vi "Core Action.vi"(8 "error in (no error)":errorcluster, 10 "SECS-II Class In":refnum<class "SECS-II Class.lvclass">, 11 "33-Update Trace Data in":refnum<class "33-Update Trace Data.lvclass">) -> (0 "error out":errorcluster, 2 "SECS-II Class Out":refnum<class "SECS-II Class.lvclass">, 3 "33-Update Trace Data out":refnum<class "33-Update Trace Data.lvclass">)   [LabVIEW 2020, in "SECS Scenarios.lvlib" / "33-Update Trace Data.lvclass"]
uses:
  33-Update Trace Data.lvclass
  D:/Dropbox/SECS/SECS_GEM v1.1.0/Com/SECS Scenarios/Scenarios Class/Scenarios Class.lvclass
  SECS Communication/SECS-II Class/SECS-II Class.lvclass
  SECS Communication/S6 Message Class/S6 Message Class.lvclass
  D:/Dropbox/SECS/SECS_GEM v1.1.0/Com/SECS Communication/SECS-II Class/SECS-II Class.lvclass
  33-Update Trace Data.lvclass/33-Update Trace Data.ctl
  Scenarios Class/Scenarios Class.lvclass/Scenarios Class.ctl
  Scenarios Class/Reply State.ctl
  Scenarios Class/Write Reply State.vi
  Scenarios Class/Read HSMS Class.vi
  SECS Communication/HSMS Class/HSMS Class.lvclass
  Scenarios Class/Scenarios Class.lvclass
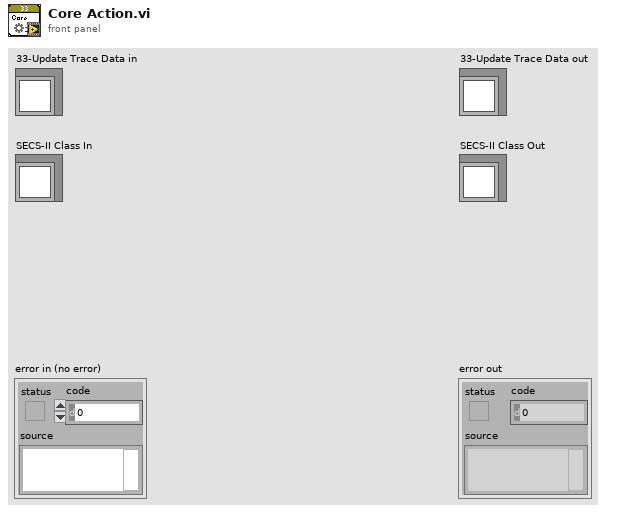
[diagram p1: front panel]
types:
  T1 = typedef "SECS Communication.lvlib/S6 Message Class.lvclass/S6F1.ctl" = cluster{"TRID":u32, "SMPLN":u32, "STIME":string, "SV":cluster{"Format Code":T2, "Value":variant}[]}
  T2 = typedef "SECS Communication.lvlib/SECS-II Class.lvclass/Format Code.ctl" = enum16{"L", "A", "B", "Boolean", "J", "I1", "I2", "I4", "I8", "U1", "U2", "U4", "U8", "F4", "F8", "Char"}
  T3 = typedef "SECS Scenarios.lvlib/Scenarios Class.lvclass/Reply State.ctl" = enum16{"OK", "Illegal Data", "Unknown Stream", "Unknown Function", "Off-Line", "T3 Timeout", "Inner-Timeout"}
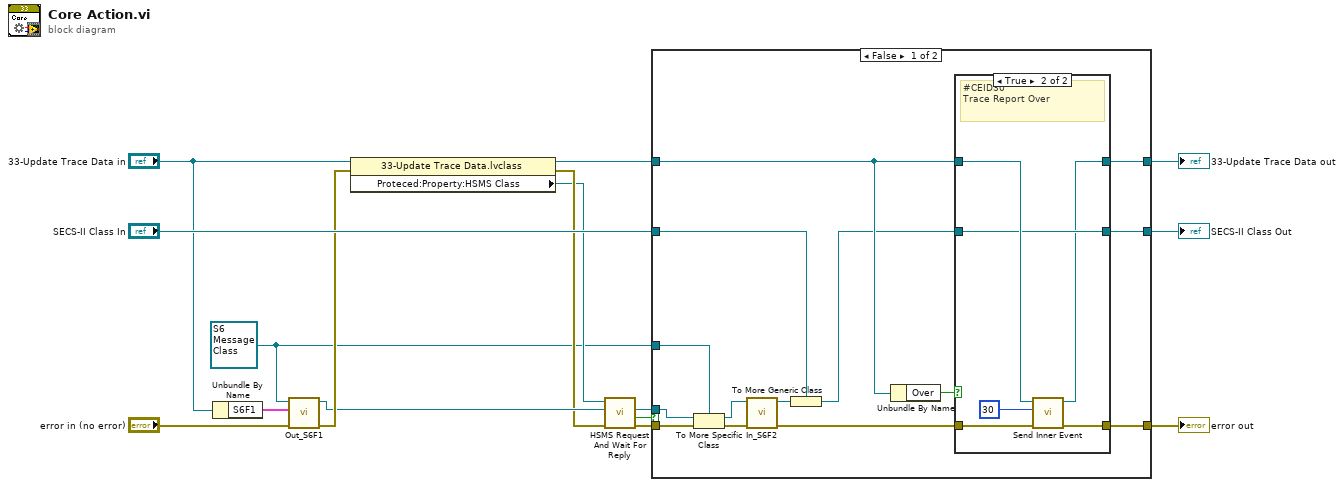
[diagram p0: block diagram]
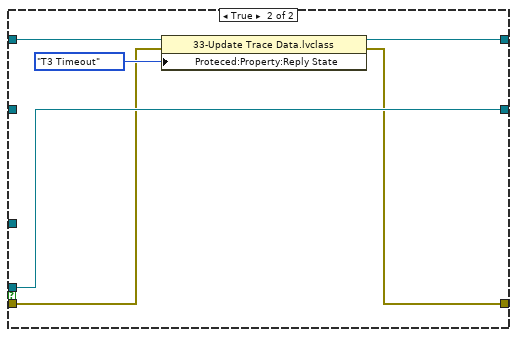
[diagram p3: hidden frame]
diagram:
  w5 = refnum<class "S6 Message Class.lvclass"> refnum ("SECS Communication.lvlib:S6 Message Class.lvclass")
  n1 = Unbundle By Name("33-Update Trace Data in") -> ("S6F1"=w4:T1)
  n2 = call "Out_S6F1.vi"("error in (no error)"="error in (no error)", "S6F1"=w4, "S6 Message Class in"=w5) -> ("error out"=w13:errorcluster, "S6 Message Class out"=w12:refnum<class "S6 Message Class.lvclass">)  [unwired: 7 in]
  n3 = property class="33-Update Trace Data.lvclass"(reference="33-Update Trace Data in", error in=w13) -> (reference out=w6:refnum<class "33-Update Trace Data.lvclass">, error out=w11:errorcluster, "Proteced:Property:HSMS Class"=w10:refnum<class "HSMS Class.lvclass">)
  n4 = call "HSMS Request And Wait For Reply.vi"("error in (no error)"=w11, "SECS-II Class In"=w12, "HSMS Class in"=w10) -> ("error out"=w9:errorcluster, "Timeout?"=w8:bool, "SECS-II Class Out"=w7:refnum<class "SECS-II Class.lvclass">)  [unwired: 5 in, 1 out]
  n5 = case shown="False" w8 {
    tunnel: w9 -> [w30 w42]
    tunnel: w7 -> [w29 w45]
    tunnel: w5 -> [w28 _]
    tunnel: w6 -> [w20 w44]
    tunnel: [w17 w41] -> w1
    tunnel: [w21 w40] -> w3
    tunnel: "SECS-II Class In" -> [w24 _]
    tunnel: [w18 w45] -> w2
    frame False {
      n6 = To More Specific Class(target class=w28, reference=w29, error in=w30) -> (specific class reference=w26:refnum<class "S6 Message Class.lvclass">, error out=w27:errorcluster)
      n7 = call "In_S6F2.vi"("error in (no error)"=w27, "S6 Message Class in"=w26) -> ("error out"=w23:errorcluster, "S6 Message Class out"=w25:refnum<class "S6 Message Class.lvclass">)  [unwired: 6 in, 2 out]
      n8 = To More Generic Class(target class=w24, reference=w25) -> (generic class reference=w19:refnum<class "SECS-II Class.lvclass">)
      n9 = Unbundle By Name(w20) -> ("Over"=w22:bool)
      n10 = case shown="True" w22 {
        tunnel: w23 -> [w33 w39]
        tunnel: [w33 w38] -> w21
        tunnel: w20 -> [w32 w37]
        tunnel: w19 -> [w31 w35]
        tunnel: [w31 w35] -> w18
        tunnel: [w32 w34] -> w17
        frame False {
        }
        frame True {
          # "#CEID30\nTrace Report Over"
          n11 = call "Send Inner Event.vi"("error in (no error)"=w39, "CEID"=u32 30, "Scenarios Class in"=w37) -> ("error out"=w38:errorcluster, "Scenarios Class out"=w34:refnum<class "33-Update Trace Data.lvclass">)  [unwired: 7 in]
        }
      }
    }
    frame True {
      n12 = property class="33-Update Trace Data.lvclass"(reference=w44, error in=w42, "Proteced:Property:Reply State"=Reply_State."T3 Timeout" ("Reply State")) -> (reference out=w41:refnum<class "33-Update Trace Data.lvclass">, error out=w40:errorcluster)
    }
  }
  "error out" <- w3
  "33-Update Trace Data out" <- w1
  "SECS-II Class Out" <- w2
